vi "InterruptMeasZ.vi"(8 "error in (no error)":errorcluster, 9 "meas_id":string[](array[string])=["1", "2", "3", "4", "5", "6", "7", "8", "9", "10"], 10 "next index":u16=1, 11 "current index":u16) -> (0 "error out":errorcluster, 1 "Select list out":string[](array[string]), 2 "new next index":u16, 3 "Interrupt after meas":bool, 4 "VI's path":string="InterruptMeasZ.vi")   [LabVIEW 2016]
doc: "Displays the list of measSetIds being measured, and allows the user to select which measurement will be run next.\n\n It is designed to be called once at the beginning of a measurement, to display the ID list, and once at the end to read any interrupts. When it is called, it displays the input ID list updated with markers showing the current measurement and next measurement. For reading interrupts, it may be called with an empty input ID list, and the displayed list doesn't change. It returns the user interrupt state and next measurement."
panel:
  in  "Interrupt after meas":bool
  in  "Select next meas":u16(ring) items=["spot check: 976", "984", "992", "1000", "1008", "1016", "1024", "current meas: end"]
  # "Program constants"
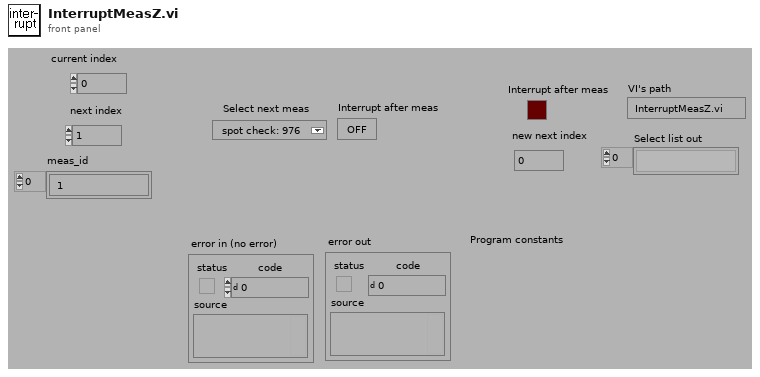
[diagram p1: front panel]
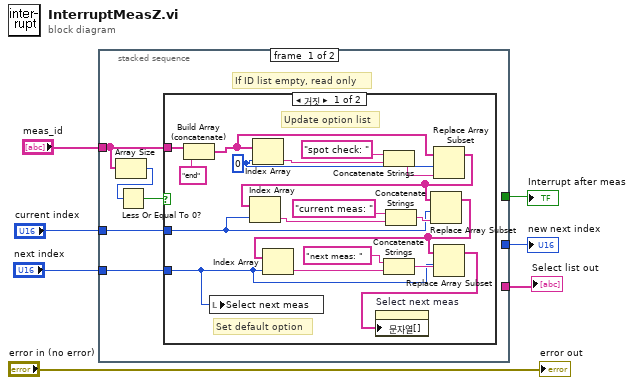
[diagram p0: block diagram]
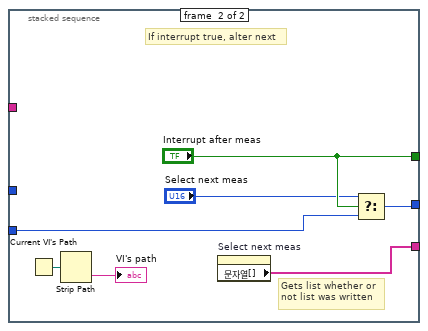
[diagram p3: hidden frame]
diagram:
  n1 = stacked-sequence {
    tunnel: "meas_id" -> [w10 _]
    tunnel: "current index" -> [w12 _]
    tunnel: "next index" -> [w11 w36]
    tunnel: [_ "Interrupt after meas"] -> w4
    tunnel: [_ w35] -> w3
    tunnel: [_ w34] -> w1
    frame #0 {
      # "If ID list empty, read only"
      n2 = Array Size(array=w10) -> (size(s)=w9:i32)
      n3 = Less Or Equal To 0?(x=w9) -> (x <= 0?=w8:bool)
      n4 = case shown="거짓" w8 {
        tunnel: w12 -> [w19 _]
        tunnel: w11 -> [w13 _]
        tunnel: w10 -> [w16 _]
        frame False {
          w21 = 0 ("index")
          # "Set default option"
          # "Update option list"
          n5 = Build Array (concatenate)(w16, "end") -> (w15:string[])
          n6 = local write "Select next meas"(w13) -> ()
          n7 = Index Array(array=w15, index=w21) -> (element=w27:string)
          n8 = Concatenate Strings("spot check: " ("Substring"), w27) -> (w24:string)
          n9 = Replace Array Subset(array=w15, new element=w24, index=w21) -> (w18:string[])
          n10 = Index Array(array=w18, index=w19) -> (element=w26:string)
          n11 = Concatenate Strings("current meas: " ("Substring"), w26) -> (w23:string)
          n12 = Replace Array Subset(array=w18, new element=w23, index=w19) -> (w17:string[])
          n13 = Index Array(array=w17, index=w13) -> (element=w25:string)
          n14 = Concatenate Strings("next meas: " ("Substring"), w25) -> (w22:string)
          n15 = Replace Array Subset(array=w17, new element=w22, index=w13) -> (w14:string[])
          n16 = property on="Select next meas" class="Ring (엄격한)"("문자열[]"=w14) -> ()  [unwired: 2 in, 2 out]
        }
        frame True {
          # "Don't alter option list"
        }
      }
    }
    frame #1 {
      # "Gets list whether or\nnot list was written"
      # "If interrupt true, alter next"
      n17 = Current VI's Path() -> (path=w32:path)
      n18 = Strip Path(path=w32) -> (name=→"VI's path":string)  [unwired: 1 out]
      n19 = property on="Select next meas" class="Ring (엄격한)"() -> ("문자열[]"=w34:string[])  [unwired: 2 in, 2 out]
      n20 = Select(t="Select next meas", s="Interrupt after meas", f=w36) -> (s? t:f=w35:u16)
    }
  }
  "new next index" <- w3
  "Interrupt after meas" <- w4
  "Select list out" <- w1
  "error out" <- "error in (no error)"
